vi "Test.vi"() -> ()   [LabVIEW 2024]
uses:
  Sample State Actor/Idle/Idle.lvclass
  C:/Users/ottoa/OneDrive/Desktop/working copies/stateActor/src/State Actor/State Actor.lvclass
  <vilib>/ActorFramework/Message Enqueuer/Message Enqueuer.lvclass/Message Enqueuer.ctl
  <vilib>/ActorFramework/Message Enqueuer/Enqueue.vi
  Sample State Actor/Main Messages/Cycle Start Msg/Cycle Start Msg.lvclass
  C:/Program Files (x86)/National Instruments/LabVIEW 2024/vi.lib/ActorFramework/Message/Message.lvclass
  Sample State Actor/Main Messages/Reset Msg/Reset Msg.lvclass
  Sample State Actor/Main Messages/Cycle Complete Msg/Cycle Complete Msg.lvclass
  <vilib>/ActorFramework/Stop Msg/Stop Msg.lvclass
  <vilib>/ActorFramework/Message Priority Queue/Priority Enqueue.vi
  State Actor/State Actor.lvclass
panel:
  out "Array":T1(array[cluster]) {"Time Stamp" format="%<%x %.3X>T"}
  in  "Reset":bool
  in  "Stop":bool
  in  "Cycle Complete":bool
  in  "Cycle Start":bool
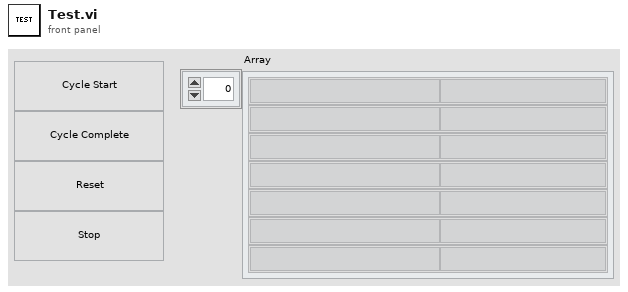
[diagram p1: front panel]
types:
  T1 = cluster{"Time Stamp":timestamp, "String":string}[]
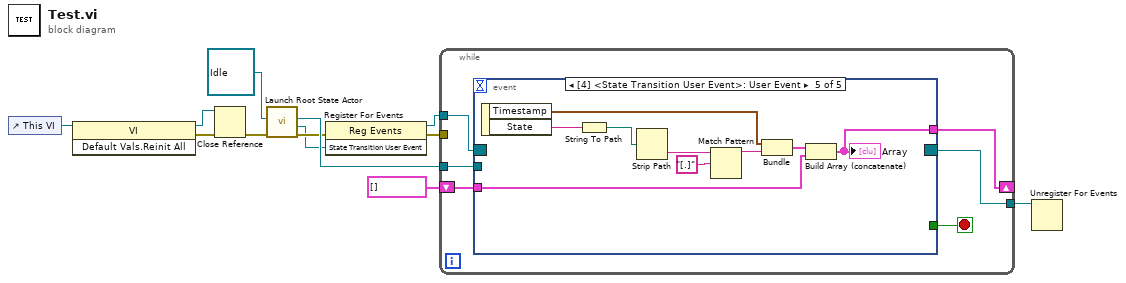
[diagram p0: block diagram]
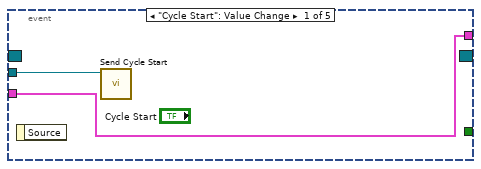
[diagram p2: hidden frame]
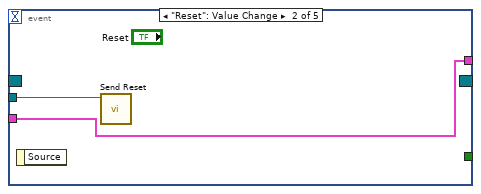
[diagram p3: hidden frame]
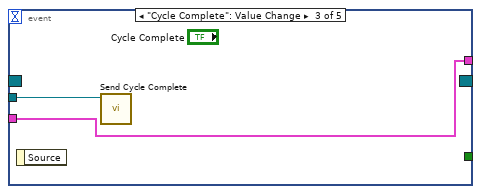
[diagram p4: hidden frame]
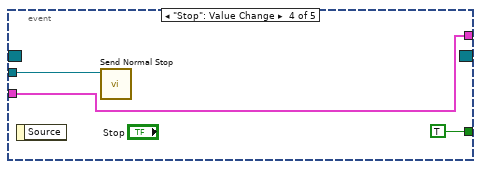
[diagram p5: hidden frame]
diagram:
  n1 = control-ref of="This VI"() -> (w10:refnum<vi>)
  n2 = invoke class="VI" method="Default Vals.Reinit All"(reference=w10) -> (reference out=w9:refnum<vi>, error out=w8:errorcluster)  [unwired: 2 in, 1 out]
  n3 = Close Reference(reference=w9, error in (no error)=w8) -> (error out=w7:errorcluster)
  n4 = call "Launch Root State Actor.vi"("error in (no error)"=w7, "State Actor"=refnum<class "Idle.lvclass"> refnum ("Sample State Actor.lvlib:Idle.lvclass")) -> ("error out"=w6:errorcluster, "State Transition User Event"=w4:refnum<user-event>, "Actor's Enqueuer"=w12:refnum<class "Message Enqueuer.lvclass">)  [unwired: 7 in]
  n5 = register-events(error in=w6, w4) -> (reference out=w3:refnum<event-registration>, error out=w5:errorcluster)  [unwired: 1 in]
  n6 = while {
    tunnel: w12 -> [w18]
    tunnel: [w16] -> w11
    shift-right: [w14] -> _
    shift-left: T1 [] ("Array") -> [w15]
    tunnel: w5 -> [_]
    tunnel: w3 -> [w13]
    stop <- w17 stop-if-true
    n7 = event shown="[4] <State Transition User Event>: User Event" {
      selector: w13 -> [_ _ _ _ _]
      dyn-events: [_ _ _ _ _] -> w16
      timeout: _ -> [_ _ _ _ _]
      tunnel: w18 -> [w20 w22 w24 w27 _]
      tunnel: [_ _ _ TRUE _] -> w17
      tunnel: w15 -> [w19 w21 w23 w25 w31]
      tunnel: [w19 w21 w23 w25 w29] -> w14
      event "Cycle Start": Value Change {
        n8 = event-data() -> ()  [unwired: 1 in, 1 out]
        n9 = call "Send Cycle Start.vi"("Message Enqueuer"=w20) -> ()  [unwired: 9 in, 2 out]
      }
      event "Reset": Value Change {
        n10 = event-data() -> ()  [unwired: 1 in, 1 out]
        n11 = call "Send Reset.vi"("Message Enqueuer"=w22) -> ()  [unwired: 9 in, 2 out]
      }
      event "Cycle Complete": Value Change {
        n12 = event-data() -> ()  [unwired: 1 in, 1 out]
        n13 = call "Send Cycle Complete.vi"("Message Enqueuer"=w24) -> ()  [unwired: 9 in, 2 out]
      }
      event "Stop": Value Change {
        n14 = event-data() -> ()  [unwired: 1 in, 1 out]
        n15 = call <vilib>:"Send Normal Stop.vi"("Message Enqueuer"=w27) -> ()  [unwired: 10 in, 1 out]
      }
      event User Event {
        n16 = event-data() -> ("Timestamp"=w33:timestamp, "State"=w28:string)  [unwired: 1 in]
        n17 = String To Path(string=w28) -> (path=w35:path)
        n18 = Strip Path(path=w35) -> (name=w36:string)  [unwired: 1 out]
        n19 = Match Pattern(string=w36, regular expression="[.]") -> (before substring=w32:string)  [unwired: 1 in, 3 out]
        n20 = Bundle("Timestamp"=w33, "name"=w32) -> (w30:cluster{"Timestamp":timestamp, "name":string})  [unwired: 1 in]
        n21 = Build Array (concatenate)(w30, w31) -> (w29:T1)
        "Array" <- w29
      }
    }
  }
  n22 = Unregister For Events(event registration refnum=w11) -> ()  [unwired: 1 in, 1 out]
